vi "Write INI.vi"(1 "Conversion and Correction":dbl[][][](array[numeric]), 2 "error in (no error)":errorcluster, 3 "Path":path) -> (0 "error out":errorcluster)   [LabVIEW 2022 SP3]
uses:
  <vilib>/Utility/config.llb/Write Key (Double).vi
  <vilib>/Utility/config.llb/NI_LVConfig.lvlib
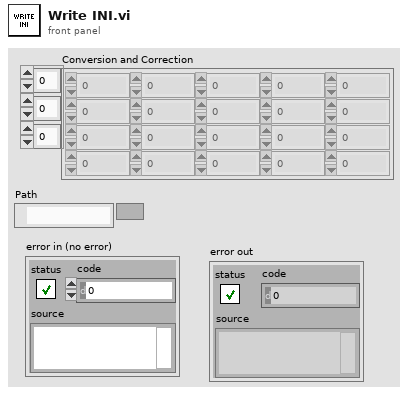
[diagram p1: front panel]
types:
  T1 = typedef "NI_LVConfig.lvlib/Config Data RefNum.ctl" = refnum<k1>
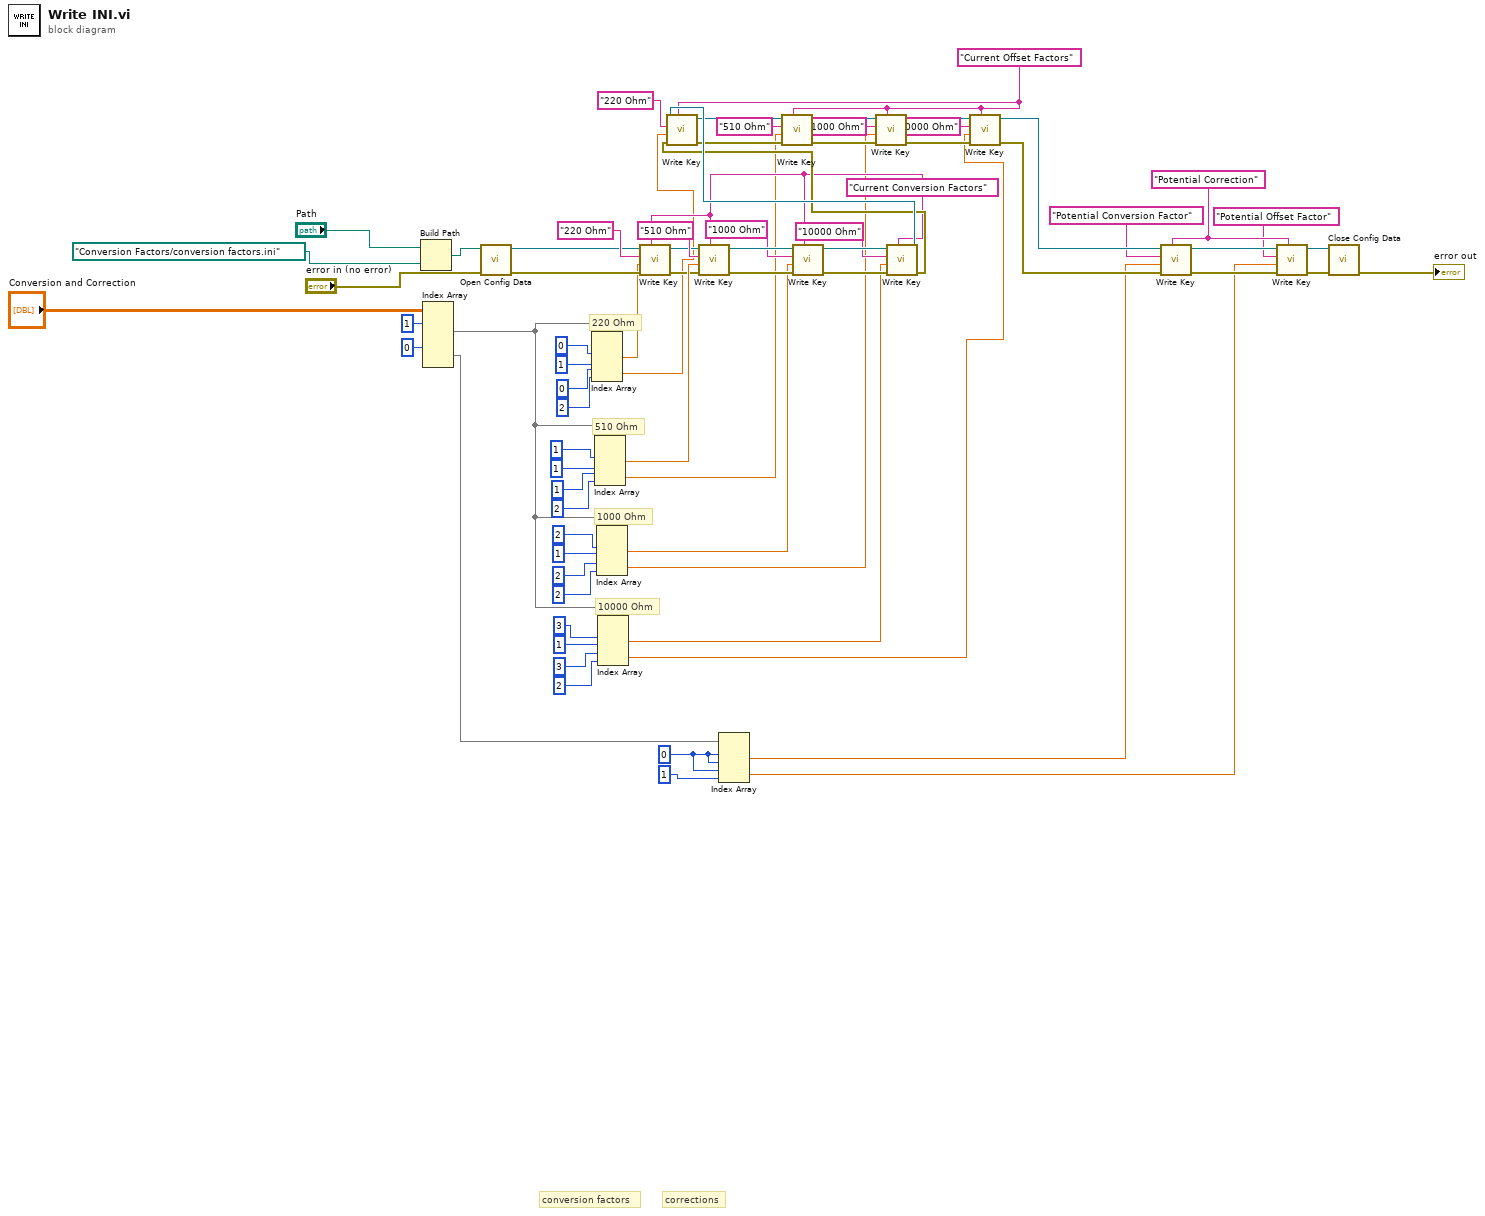
[diagram p0: block diagram]
diagram:
  w3 = "Potential Correction" ("section")
  w7 = 0 ("index (row)")
  w31 = "Current Offset Factors" ("section")
  w35 = "Current Conversion Factors" ("section")
  # "220 Ohm"
  # "corrections"
  # "conversion factors"
  # "10000 Ohm"
  # "1000 Ohm"
  # "510 Ohm"
  n1 = Build Path(base path="Path", name or relative path=path "Conversion Factors/conversion factors.ini") -> (appended path=w53:path)
  n2 = Index Array(array="Conversion and Correction", index (dim 0) #1=1 ("index (page)"), index (dim 0) #2=0 ("index (page)")) -> (element #1=w28:dbl[][], element #2=w14:dbl[][])  [unwired: 4 in]
  n3 = call <vilib>:"Open Config Data.vi"("error in (no error)"="error in (no error)", "configuration file path"=w53) -> ("error out"=w42:errorcluster, "refnum"=w41:T1)  [unwired: 7 in, 1 out]
  n4 = Index Array(array=w28, index (row) #1=0 ("index (row)"), index (col) #1=1 ("disabled index (col)"), index (row) #2=0 ("index (row)"), index (col) #2=2 ("disabled index (col)")) -> (element #1=w36:dbl, element #2=w25:dbl)
  n5 = Index Array(array=w28, index (row) #1=1 ("index (row)"), index (col) #1=1 ("disabled index (col)"), index (row) #2=1 ("index (row)"), index (col) #2=2 ("disabled index (col)")) -> (element #1=w57:dbl, element #2=w22:dbl)
  n6 = Index Array(array=w28, index (row) #1=2 ("index (row)"), index (col) #1=1 ("disabled index (col)"), index (row) #2=2 ("index (row)"), index (col) #2=2 ("disabled index (col)")) -> (element #1=w56:dbl, element #2=w19:dbl)
  n7 = Index Array(array=w28, index (row) #1=3 ("index (row)"), index (col) #1=1 ("disabled index (col)"), index (row) #2=3 ("index (row)"), index (col) #2=2 ("disabled index (col)")) -> (element #1=w55:dbl, element #2=w16:dbl)
  n8 = call-poly <vilib>:"Write Key.vi"("section"=w35, "error in (no error)"=w42, "value"=w36, "key"="220 Ohm", "refnum"=w41) -> ("error out"=w39:errorcluster, "refnum out"=w40:T1)  [unwired: 4 in, 1 out]
  n9 = call-poly <vilib>:"Write Key.vi"("section"=w35, "error in (no error)"=w39, "value"=w57, "key"="510 Ohm", "refnum"=w40) -> ("error out"=w63:errorcluster, "refnum out"=w67:T1)  [unwired: 4 in, 1 out]
  n10 = Index Array(array=w14, index (row) #1=w7, index (col) #1=w7, index (row) #2=w7, index (col) #2=1 ("index (row)")) -> (element #1=w5:dbl, element #2=w4:dbl)
  n11 = call-poly <vilib>:"Write Key.vi"("section"=w35, "error in (no error)"=w63, "value"=w56, "key"="1000 Ohm", "refnum"=w67) -> ("error out"=w62:errorcluster, "refnum out"=w66:T1)  [unwired: 4 in, 1 out]
  n12 = call-poly <vilib>:"Write Key.vi"("section"=w35, "error in (no error)"=w62, "value"=w55, "key"="10000 Ohm", "refnum"=w66) -> ("error out"=w61:errorcluster, "refnum out"=w65:T1)  [unwired: 4 in, 1 out]
  n13 = call-poly <vilib>:"Write Key.vi"("section"=w31, "error in (no error)"=w61, "value"=w25, "key"="220 Ohm", "refnum"=w65) -> ("error out"=w32:errorcluster, "refnum out"=w33:T1)  [unwired: 4 in, 1 out]
  n14 = call-poly <vilib>:"Write Key.vi"("section"=w31, "error in (no error)"=w32, "value"=w22, "key"="510 Ohm", "refnum"=w33) -> ("error out"=w45:errorcluster, "refnum out"=w46:T1)  [unwired: 4 in, 1 out]
  n15 = call-poly <vilib>:"Write Key.vi"("section"=w31, "error in (no error)"=w45, "value"=w19, "key"="1000 Ohm", "refnum"=w46) -> ("error out"=w44:errorcluster, "refnum out"=w47:T1)  [unwired: 4 in, 1 out]
  n16 = call-poly <vilib>:"Write Key.vi"("section"=w31, "error in (no error)"=w44, "value"=w16, "key"="10000 Ohm", "refnum"=w47) -> ("error out"=w10:errorcluster, "refnum out"=w13:T1)  [unwired: 4 in, 1 out]
  n17 = call-poly <vilib>:"Write Key.vi"("section"=w3, "error in (no error)"=w10, "value"=w5, "key"="Potential Conversion Factor", "refnum"=w13) -> ("error out"=w9:errorcluster, "refnum out"=w12:T1)  [unwired: 4 in, 1 out]
  n18 = call-poly <vilib>:"Write Key.vi"("section"=w3, "error in (no error)"=w9, "value"=w4, "key"="Potential Offset Factor", "refnum"=w12) -> ("error out"=w8:errorcluster, "refnum out"=w11:T1)  [unwired: 4 in, 1 out]
  n19 = call <vilib>:"Close Config Data.vi"("error in (no error)"=w8, "refnum"=w11) -> ("error out"=→"error out":errorcluster)  [unwired: 8 in, 1 out]
